vi "Open folder in new window.vi"(8 "error in (no error)":errorcluster, 11 "Directory to open":path) -> (0 "error out":errorcluster)   [LabVIEW 2020]
uses:
  Typedefs/Set Main VI cursor.ctl
  Global Variables/General Globals.vi
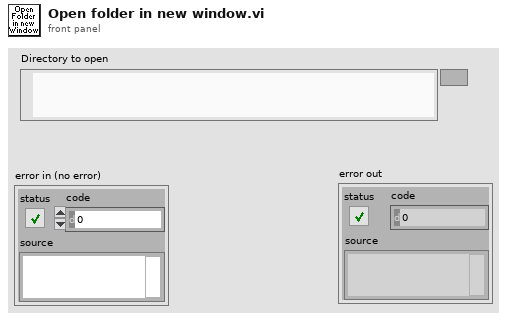
[diagram p1: front panel]
types:
  T1 = typedef "Set Main VI cursor.ctl" = enum16{"Release busy cursor", "Set busy cursor"}
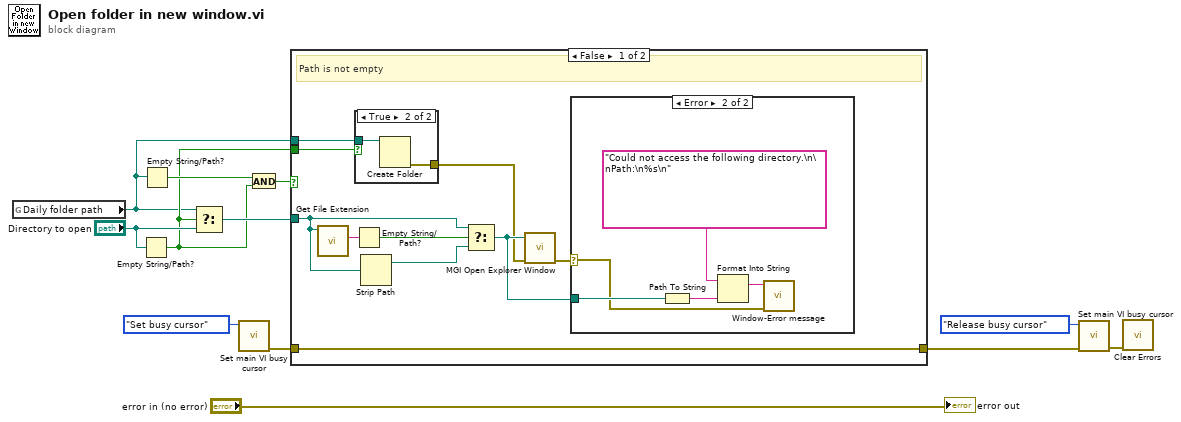
[diagram p0: block diagram]
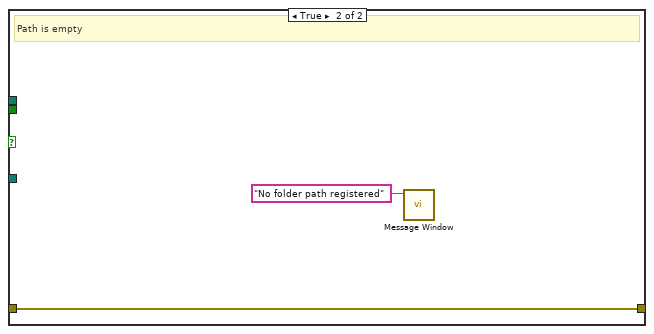
[diagram p4: hidden frame]
diagram:
  n1 = global read "General Globals.vi" "Daily folder path"() -> (w1:path)
  n2 = Empty String/Path?(string/path="Directory to open") -> (empty?=w2:bool)
  n3 = Empty String/Path?(string/path=w1) -> (empty?=w4:bool)
  n4 = Select(t=w1, s=w2, f="Directory to open") -> (s? t:f=w5:path)
  n5 = call "Set main VI busy cursor.vi"("Main VI's cursor"=Set_Main_VI_cursor."Set busy cursor") -> ("error out"=w11:errorcluster)  [unwired: 10 in]
  n6 = And(x=w4, y=w2) -> (x .and. y?=w3:bool)
  n7 = case shown="False" w3 {
    tunnel: w5 -> [w18 _]
    tunnel: w11 -> [w16 w30]
    tunnel: [w16 w30] -> w8
    tunnel: w2 -> [w15 _]
    tunnel: w1 -> [w14 _]
    frame False {
      # "Path is not empty"
      n8 = call <vilib>:"Get File Extension.vi"("file"=w18) -> ("lowercase file extension"=w21:string)  [unwired: 6 in, 4 out]
      n9 = Empty String/Path?(string/path=w21) -> (empty?=w20:bool)
      n10 = case shown="True" w15 {
        tunnel: w14 -> [_ w24]
        tunnel: [_ w23] -> w13
        frame False {
        }
        frame True {
          n11 = Create Folder(path (use dialog)=w24) -> (error out=w23:errorcluster)  [unwired: 2 in, 2 out]
        }
      }
      n12 = Strip Path(path=w18) -> (stripped path=w19:path)  [unwired: 1 out]
      n13 = Select(t=w18, s=w20, f=w19) -> (s? t:f=w17:path)
      n14 = call <userlib>:"MGI Open Explorer Window.vi"("error in (no error)"=w13, "Directory or File"=w17) -> ("error out"=w22:errorcluster)  [unwired: 9 in]
      n15 = case shown="Error" w22 {
        selector: w22 -> [_ w25]
        tunnel: w17 -> [_ w28]
        frame No Error {
        }
        frame Error {
          n16 = Path To String(path=w28) -> (string=w27:string)
          n17 = Format Into String(format string="Could not access the following directory.\n\nPath:\n%s\n" ("Error Source"), w27) -> (resulting string=w26:string)  [unwired: 2 in, 1 out]
          n18 = call "Window-Error message.vi"("error in (no error)"=w25, "Message"=w26) -> ()  [unwired: 9 in, 1 out]
        }
      }
    }
    frame True {
      # "Path is empty"
      n19 = call "Message Window.vi"("Message string"="No folder path registered" ("Error Source")) -> ()  [unwired: 10 in, 1 out]
    }
  }
  n20 = call "Set main VI busy cursor.vi"("error in (no error)"=w8, "Main VI's cursor"=Set_Main_VI_cursor."Release busy cursor") -> ("error out"=w7:errorcluster)  [unwired: 9 in]
  n21 = call <vilib>:"Clear Errors.vi"("error in (no error)"=w7) -> ()  [unwired: 5 in, 2 out]
  "error out" <- "error in (no error)"
